vi "Add Context Menu Break.vi"(0 "NotifyIcon in":refnum<class "NotifyIcon.lvclass">, 5 "Item Tag":string, 9 "Parent Item Tag (\"\")":string, 11 "error in (no error)":errorcluster, 12 "Item Index (Last)":i32=-1) -> (4 "NotifyIcon out":refnum<class "NotifyIcon.lvclass">, 6 "dub Item Tag":string, 15 "error out":errorcluster)   [LabVIEW 2016, in "NotifyIcon.lvclass"]
doc: "This VI adds a horizontal break line to the menu. A horizontal line serves the purpose of dividing or grouping menu items into related groups for a better overview.\n\n<b>Item Tag</b>\nMust be a unique string that identifies the menu item in the item hierarchy. If this input is left empty the item will not be added to the menu.\n\n<b>Parent Item Tag</b>\nIs used to specify the Tag of the menu item that this item should refer to as its parent. Leaving this input empty or unwired will insert the menu item at the menu root.\n\n<b>Item Index</b>\nWire this input to a numeric value to insert menu items in the middel or top of the menu. Leaving the input unwired inserts the item as the last element under the specified branch (default -1).\n\n\nStinus Olsen\nCIM Industrial Systems A/S\n22. Feb. 2011 15:03\nmailto: seo@cim.as"
uses:
  NotifyIcon.lvclass
  NotifyIcon.lvclass/NotifyIcon.ctl
  System.Windows.Forms
panel:
  # "This VI belongs to the NotifyIcon Toolset. \nA toolset that makes it easy to create, control and manipulate a notification icon in the notification area of the Windows taskbar.\nThe toolset requires Microsoft .NET framework 2.0\n\n\nNOTICE -- YOU MUST LEAVE THIS NOTICE IN PLACE.  PER THE TERMS OF THE LICENSE BELOW, YOU MAY SUBLICENSE THIS SOFTWARE \nIN ANY WAY THAT DOES NOT CONFLICT WITH THIS LICENSE.\n\n### BSD License (http://www.opensource.org/licenses/bsd-license.php) Begin ###\n \nCopyright (c) 2011, Stinus Olsen <seo@cim.as>\n\nAll rights reserved.\n\nRedistribution and use in source and binary forms, with or without modification, are permitted provided that the following conditions are met:\n\n    * Redistributions of source code must retain the above copyright notice, this list of conditions and the following disclaimer.\n    * Redistributions in binary form must reproduce the above copyright notice, this list of conditions and the following disclaimer in the \n       documentation and/or other materials provided with the distribution.\n    * Neither the name of CIM Industrial Systems nor the names of its contributors may be used to endorse or promote products derived \n       from this software without specific prior written permission.\n\nTHIS SOFTWARE IS PROVIDED BY THE COPYRIGHT HOLDERS AND CONTRIBUTORS \"AS IS\" AND ANY EXPRESS OR IMPLIED WARRANTIES, \nINCLUDING, BUT NOT LIMITED TO, THE IMPLIED WARRANTIES OF MERCHANTABILITY AND FITNESS FOR A PARTICULAR PURPOSE ARE \nDISCLAIMED. IN NO EVENT SHALL THE COPYRIGHT OWNER OR CONTRIBUTORS BE LIABLE FOR ANY DIRECT, INDIRECT, INCIDENTAL,\n SPECIAL, EXEMPLARY, OR CONSEQUENTIAL DAMAGES (INCLUDING, BUT NOT LIMITED TO, PROCUREMENT OF SUBSTITUTE GOODS OR \nSERVICES; LOSS OF USE, DATA, OR PROFITS; OR BUSINESS INTERRUPTION) HOWEVER CAUSED AND ON ANY THEORY OF LIABILITY, \nWHETHER IN CONTRACT, STRICT LIABILITY, OR TORT (INCLUDING NEGLIGENCE OR OTHERWISE) ARISING IN ANY WAY OUT OF THE USE \nOF THIS SOFTWARE, EVEN IF ADVISED OF THE POSSIBILITY OF SUCH DAMAGE.\n\n### BSD License End ###"
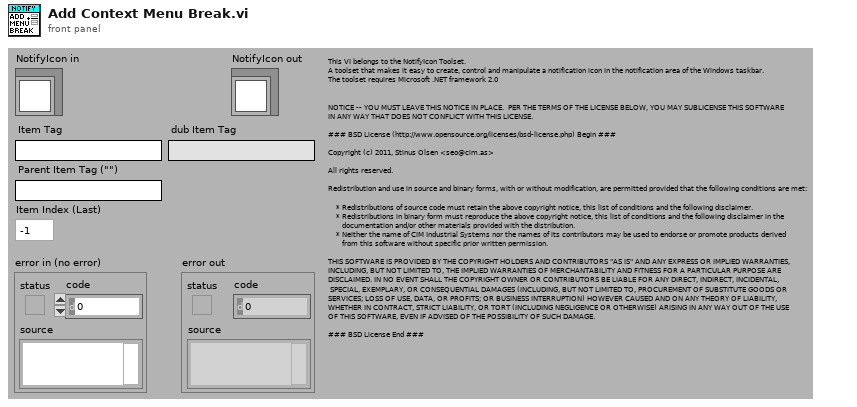
[diagram p1: front panel]
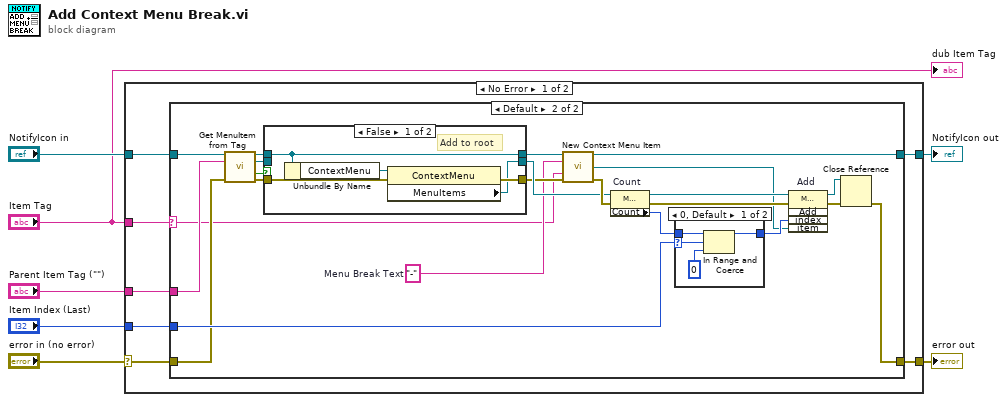
[diagram p0: block diagram]
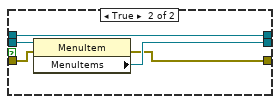
[diagram p3: hidden frame]
diagram:
  n1 = case shown="No Error" "error in (no error)" {
    selector: "error in (no error)" -> [w10 w56]
    tunnel: [w14 w56] -> w6
    tunnel: [w9 w55] -> w4
    tunnel: "NotifyIcon in" -> [w12 w55]
    tunnel: "Parent Item Tag (\"\")" -> [w11 _]
    tunnel: "Item Tag" -> [w8 _]
    tunnel: "Item Index (Last)" -> [w13 _]
    frame No Error {
      n2 = case shown="Default" w8 {
        selector: w8 -> [_ w17]
        tunnel: [w15 w39] -> w14
        tunnel: w13 -> [_ w38]
        tunnel: w12 -> [w16 w37]
        tunnel: w11 -> [_ w36]
        tunnel: w10 -> [w15 w35]
        tunnel: [w16 w20] -> w9
        frame "" {
        }
        frame Default {
          w18 = "-"  # Menu Break Text
          n3 = call "Get MenuItem from Tag.vi"("NotifyIcon in"=w37, "Item Tag"=w36, "error in (no error)"=w35) -> ("NotifyIcon out"=w26:refnum<class "NotifyIcon.lvclass">, "MenuItem"=w23:refnum<k24>, "Found"=w25:bool, "error out"=w24:errorcluster)  [unwired: 9 out]
          n4 = case shown="False" w25 {
            tunnel: w26 -> [w43 w49]
            tunnel: [w43 w49] -> w19
            tunnel: w24 -> [w42 w46]
            tunnel: w23 -> [_ w47]
            tunnel: [w40 w48] -> w22
            tunnel: [w41 w45] -> w21
            frame False {
              # "Add to root"
              n5 = Unbundle By Name(w43) -> ("ContextMenu"=w44:refnum<k24>)
              n6 = property class="ContextMenu"(reference=w44, error in=w42) -> (error out=w41:errorcluster, "MenuItems"=w40:refnum<k24>)  [unwired: 1 out]
            }
            frame True {
              n7 = property class="MenuItem"(reference=w47, error in=w46) -> (error out=w45:errorcluster, "MenuItems"=w48:refnum<k24>)  [unwired: 1 out]
            }
          }
          n8 = call "New Context Menu Item.vi"("NotifyIcon in"=w19, "MenuItem Text"=w18, "MenuItem Tag"=w17, "error in (no error)"=w21) -> ("dub NotifyIcon"=w20:refnum<class "NotifyIcon.lvclass">, "MenuItem"=w27:refnum<k24>, "error out"=w28:errorcluster)  [unwired: 9 out]
          n9 = property on="Count" class="Menu+MenuItemCollection"(reference=w22, error in=w28) -> (reference out=w32:refnum<k24>, error out=w31:errorcluster, "Count"=w34:i32)
          n10 = case shown="0, Default" w38 {
            selector: w38 -> [w53 _]
            tunnel: w34 -> [w52 w54]
            tunnel: [w50 w54] -> w33
            frame 0, Default {
              n11 = In Range and Coerce(upper limit=w52, x=w53, lower limit=0) -> (coerced(x)=w50:i32)  [unwired: 1 out]
            }
            frame ..-1 {
            }
          }
          n12 = invoke on="Add" class="Menu+MenuItemCollection" method="Add"(reference=w32, error in=w31, "index"=w33, "item"=w27) -> (reference out=w29:refnum<k24>, error out=w30:errorcluster)  [unwired: 1 in, 3 out]
          n13 = Close Reference(reference=w29, error in (no error)=w30) -> (error out=w39:errorcluster)
        }
      }
    }
    frame Error {
    }
  }
  "error out" <- w6
  "NotifyIcon out" <- w4
  "dub Item Tag" <- "Item Tag"
